vi "Init.vi"(8 "Error In":errorcluster, 10 "Data":variant) -> (0 "Error Out":errorcluster)   [LabVIEW 2015, in "Entry Console.lvlib"]
doc: "VI used to call initial state in this module."
uses:
  Entry Console.lvlib
  Private Controls/Module Data Cluster.ctl
  Private Controls/Module Action.ctl
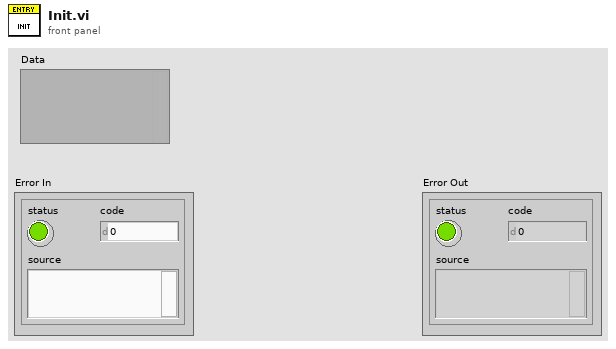
[diagram p1: front panel]
types:
  T1 = typedef "Entry Console.lvlib/Module Data Cluster.ctl" = cluster{"Data":variant, "Action":T2}
  T2 = typedef "Entry Console.lvlib/Module Action.ctl" = enum16{"Init", "Close", "Error", "Start Wash"}
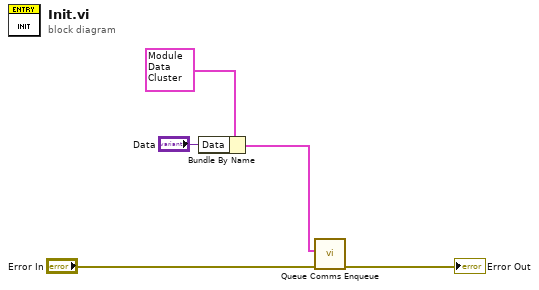
[diagram p0: block diagram]
diagram:
  n1 = Bundle By Name(cluster=T1 {"Data"=variant, "Action"=enum."Init"} ("Message Data"), "Data"="Data") -> (w3:T1)
  n2 = call "Queue Comms Enqueue.vi"("Error In"="Error In", "Message Data"=w3) -> ("Error Out"=→"Error Out":errorcluster)  [unwired: 9 in]
